vi "Calculo_conversao_4096_to_or_from_Max_Min.vi"(8 "Tipo":enum16{"Saida", "Entrada"}(ring), 9 "Min":dbl, 10 "Max":dbl, 11 "Value":variant) -> (3 "Value 2":variant)   [LabVIEW 2019]
uses:
  <vilib>/Utility/Data Type/NI_Data Type.lvlib
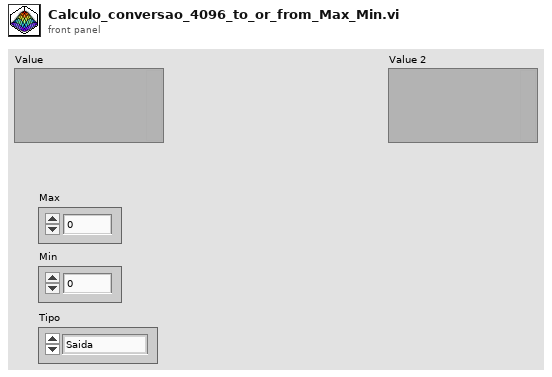
[diagram p1: front panel]
types:
  T1 = typedef "NI_Data Type.lvlib/Data Type.ctl" = enum8{"Invalid Type", "Void", "I8", "I16", "I32", "I64", "U8", "U16", "U32", "U64", "Single Float", "Double Float", "Extended Float", "Single Complex", "Double Complex", "Extended Complex", "Enum U8", "Enum U16", "Enum U32", "Enum U64", "Single Float With Unit", "Double Float With Unit", "Extended Float With Unit", "Single Complex with Unit", "Double Complex with Unit", "Extended Complex with Unit", "Boolean", "String", "Path", "Picture", "Tag", "Array", "Cluster", "Variant", "LV Variant", "Waveform", "Timestamp", "Digital Waveform", "Digital Data", "ExpressData", "Refnum", "External Data", "VI", "Poly VI", "LabVIEW Class Instance", "Fixed Point", "Set Collection", "Map Collection"}
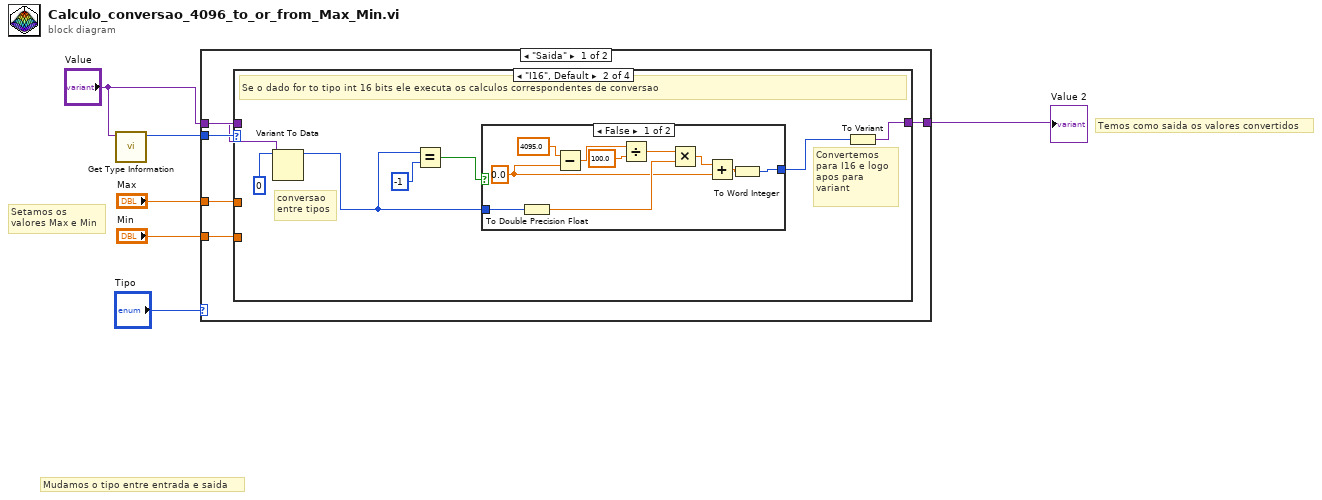
[diagram p0: block diagram]
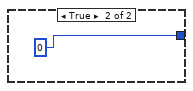
[diagram p3: hidden frame]
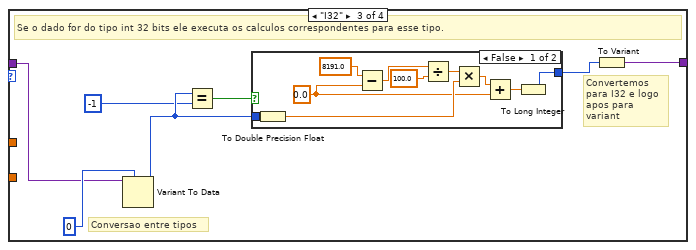
[diagram p4: hidden frame]
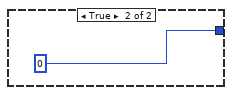
[diagram p5: hidden frame]
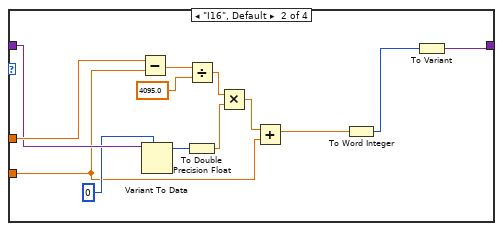
[diagram p9: hidden frame]
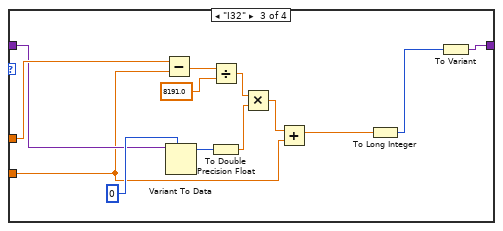
[diagram p10: hidden frame]
diagram:
  # "Temos como saida os valores convertidos"
  # "Mudamos o tipo entre entrada e saida"
  # "Setamos os valores Max e Min"
  n1 = call <vilib>:"Get Type Information.vi"("variant"="Value") -> ("type"=w5:T1)  [unwired: 6 in, 4 out]
  n2 = case shown="\"Saida\"" "Tipo" {
    tunnel: "Value" -> [w10 w50]
    tunnel: w5 -> [w11 w54]
    tunnel: "Max" -> [w8 w53]
    tunnel: "Min" -> [w7 w52]
    tunnel: [w9 w51] -> w1
    frame "Saida" {
      n3 = case shown="\"I16\", Default" w11 {
        tunnel: [w12 w17 w34 w49] -> w9
        tunnel: w8 -> [_ _ _ _]
        tunnel: w7 -> [_ _ _ _]
        tunnel: w10 -> [w12 w19 w35 w49]
        frame "Invalid Type" {
          # "Se o dado for do tipo invalido. ele apenas retorna o proprio valor"
        }
        frame "I16", Default {
          # "Convertemos para I16 e logo apos para variant"
          # "conversao entre tipos"
          # "Se o dado for to tipo int 16 bits ele executa os calculos correspondentes de conversao"
          n4 = Variant To Data(type=i16 0, Variant=w19) -> (data=w15:i16)  [unwired: 1 in, 1 out]
          n5 = Equal?(x=w15, y=i16 -1) -> (x = y?=w14:bool)
          n6 = case shown="False" w14 {
            tunnel: w15 -> [w26 _]
            tunnel: [w21 i16 0] -> w16
            frame False {
              w20 = 0.0
              n7 = To Double Precision Float(number=w26) -> (double precision float=w27:dbl)
              n8 = Subtract(x=4095.0, y=w20) -> (x-y=w29:dbl)
              n9 = Divide(x=w29, y=100.0) -> (x/y=w28:dbl)
              n10 = Multiply(x=w28, y=w27) -> (x*y=w25:dbl)
              n11 = Add(x=w25, y=w20) -> (x+y=w24:dbl)
              n12 = To Word Integer(number=w24) -> (16bit integer=w21:i16)
            }
            frame True {
            }
          }
          n13 = To Variant(anything=w16) -> (Variant=w17:variant)
        }
        frame "I32" {
          # "Convertemos para I32 e logo apos para variant"
          # "Conversao entre tipos"
          # "Se o dado for do tipo int 32 bits ele executa os calculos correspondentes para esse tipo."
          n14 = Variant To Data(type=i16 0, Variant=w35) -> (data=w33:i16)  [unwired: 1 in, 1 out]
          n15 = Equal?(x=w33, y=i16 -1) -> (x = y?=w32:bool)
          n16 = case shown="False" w32 {
            tunnel: [w42 0] -> w37
            tunnel: w33 -> [w38 _]
            frame False {
              w39 = 0.0 ("y")
              n17 = To Double Precision Float(number=w38) -> (double precision float=w45:dbl)
              n18 = Subtract(x=8191.0, y=w39) -> (x-y=w47:dbl)
              n19 = Divide(x=w47, y=100.0) -> (x/y=w46:dbl)
              n20 = Multiply(x=w46, y=w45) -> (x*y=w44:dbl)
              n21 = Add(x=w44, y=w39) -> (x+y=w43:dbl)
              n22 = To Long Integer(number=w43) -> (32bit integer=w42:i32)
            }
            frame True {
            }
          }
          n23 = To Variant(anything=w37) -> (Variant=w34:variant)
        }
        frame "Double Float" {
          # "Se o dado for do tipo double float ele apenas retorna o valor"
        }
      }
    }
    frame "Entrada", Default {
      n24 = case shown="\"Double Float\"" w54 {
        tunnel: [w55 w57 w69 w82] -> w51
        tunnel: w53 -> [_ w68 w72 _]
        tunnel: w52 -> [_ w59 w70 _]
        tunnel: w50 -> [w55 w64 w71 w82]
        frame "Invalid Type" {
        }
        frame "I16", Default {
          n25 = Subtract(x=w68, y=w59) -> (x-y=w67:dbl)
          n26 = Variant To Data(type=i16 0, Variant=w64) -> (data=w61:i16)  [unwired: 1 in, 1 out]
          n27 = Divide(x=w67, y=4095.0) -> (x/y=w65:dbl)
          n28 = To Double Precision Float(number=w61) -> (double precision float=w62:dbl)
          n29 = Multiply(x=w65, y=w62) -> (x*y=w60:dbl)
          n30 = Add(x=w60, y=w59) -> (x+y=w58:dbl)
          n31 = To Word Integer(number=w58) -> (16bit integer=w56:i16)
          n32 = To Variant(anything=w56) -> (Variant=w57:variant)
        }
        frame "I32" {
          n33 = Subtract(x=w72, y=w70) -> (x-y=w81:dbl)
          n34 = Variant To Data(type=i16 0, Variant=w71) -> (data=w78:i16)  [unwired: 1 in, 1 out]
          n35 = Divide(x=w81, y=8191.0) -> (x/y=w80:dbl)
          n36 = To Double Precision Float(number=w78) -> (double precision float=w79:dbl)
          n37 = Multiply(x=w80, y=w79) -> (x*y=w77:dbl)
          n38 = Add(x=w77, y=w70) -> (x+y=w76:dbl)
          n39 = To Long Integer(number=w76) -> (32bit integer=w75:i32)
          n40 = To Variant(anything=w75) -> (Variant=w69:variant)
        }
        frame "Double Float" {
        }
      }
    }
  }
  "Value 2" <- w1
